vi "WaveformComponent, Append Duplicates.vi"(0 "waveform":waveform(dbl)={"t0"=timestamp(3474820848.0780005 s since 1904-01-01), "dt"=nan, "Y"=[]}, 1 "duplicates":i32 min=0 step=1) -> (3 "waveform out":waveform(dbl)={"t0"=timestamp(-9593225999.921999 s since 1904-01-01), "dt"=nan, "Y"=[]})   [LabVIEW 2010]
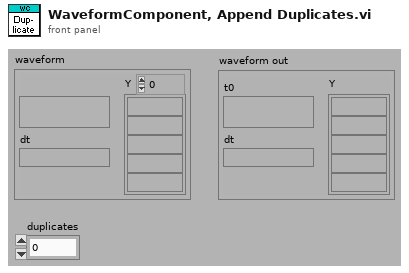
[diagram p1: front panel]
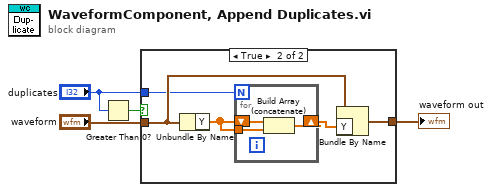
[diagram p0: block diagram]
diagram:
  n1 = Greater Than 0?(x="duplicates") -> (x > 0?=w2:bool)
  n2 = case shown="True" w2 {
    tunnel: [w5 w10] -> w4
    tunnel: "waveform" -> [w5 w7]
    tunnel: "duplicates" -> [_ w6]
    frame False {
    }
    frame True {
      n3 = Unbundle By Name(w7) -> ("Y"=w9:dbl[])
      n4 = for {
        N: w6 -> [_]
        shift-right: [w12] -> w8
        shift-left: w9 -> [w13]
        tunnel: w9 -> [w11]
        n5 = Build Array (concatenate)(w13, w11) -> (w12:dbl[])
      }
      n6 = Bundle By Name(cluster=w7, "Y"=w8) -> (w10:waveform(dbl))
    }
  }
  "waveform out" <- w4
